vi "Query_ResonantFrequency_Sub_VI.vi"(9 "error in (no error)":errorcluster, 11 "connection ID":refnum<k5>) -> (0 "error out":errorcluster, 2 "connection ID_out":refnum<k5>, 3 "Resonant Frequencies":string)   [LabVIEW 2017]
panel:
  # "OUTPUT"
  # "INPUT"
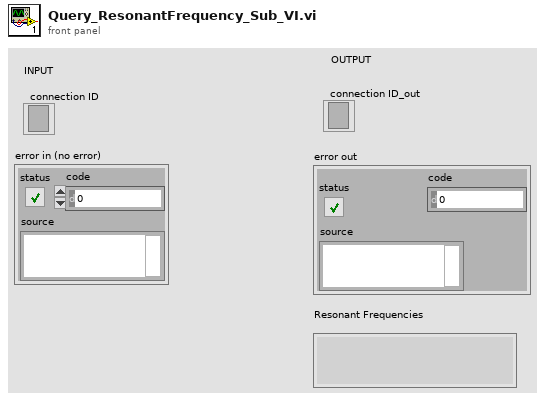
[diagram p1: front panel]
types:
  T1 = enum16{"Standard", "Buffered", "CRLF", "Immediate"}
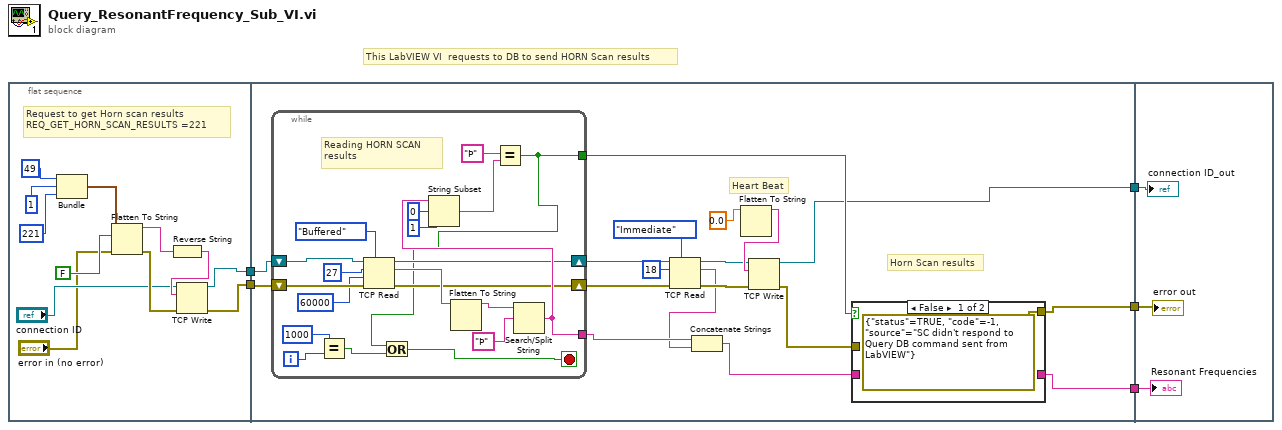
[diagram p0: block diagram]
diagram:
  # "This LabVIEW VI  requests to DB to send HORN Scan results"
  n1 = flat-sequence {
    tunnel: [w8] -> w2
    tunnel: [w7] -> w1
    tunnel: w2 -> [w33]
    tunnel: w1 -> [w32]
    tunnel: [w35] -> w5
    tunnel: [w34] -> w4
    tunnel: [w18] -> w3
    tunnel: w5 -> [w60]
    tunnel: w4 -> [w61]
    tunnel: w3 -> [w59]
    frame #0 {
      # "Request to get Horn scan results\nREQ_GET_HORN_SCAN_RESULTS =221"
      n2 = Bundle(i8 49, 1, 221) -> (w13:cluster{i8, i32, i32})  [unwired: 1 in]
      n3 = Flatten To String(anything=w13, prepend array or string size? (T)=FALSE, error in (no error)="error in (no error)") -> (data string=w12:string, error out=w16:errorcluster)  [unwired: 1 in, 1 out]
      n4 = Reverse String(1:w12) -> (0:w11:string)
      n5 = TCP Write(connection ID="connection ID", data in=w11, error in (no error)=w16) -> (connection ID out=w8:refnum<k5>, error out=w7:errorcluster)  [unwired: 1 in, 1 out]
    }
    frame #1 {
      # "Heart Beat"
      # "Horn Scan results"
      n6 = while {
        tunnel: [w37] -> w31
        tunnel: [w46] -> w21
        shift-right: [w45] -> w27
        shift-left: w33 -> [w55]
        shift-right: [w44] -> w25
        shift-left: w32 -> [w54]
        i -> [w40]
        stop <- w36 stop-if-true
        # "Reading HORN SCAN \nresults"
        n7 = Equal?(x=1000, y=w40) -> (x = y?=w38:bool)
        n8 = TCP Read(connection ID=w55, bytes to read=27, error in (no error)=w54, 7:T1."Buffered" ("mode (standard)"), 9:60000 ("timeout ms (25000)")) -> (connection ID out=w45:refnum<k5>, data out=w53:string, error out=w44:errorcluster)
        n9 = Flatten To String(anything=w53) -> (data string=w52:string)  [unwired: 3 in, 2 out]
        n10 = Search/Split String(string=w52, search string/char (-)="Þ") -> (match + rest of string=w46:string)  [unwired: 1 in, 2 out]
        n11 = String Subset(string=w46, offset (0)=0, length (rest)=1 ("length (rest)")) -> (substring=w47:string)
        n12 = Equal?(x="Þ" ("search string/char (-)"), y=w47) -> (x = y?=w37:bool)
        n13 = Or(x=w37, y=w38) -> (x .or. y?=w36:bool)
      }
      n14 = TCP Read(connection ID=w27, bytes to read=18, error in (no error)=w25, 7:T1."Immediate" ("mode (standard)")) -> (connection ID out=w26:refnum<k5>, data out=w20:string, error out=w24:errorcluster)  [unwired: 1 in]
      n15 = Concatenate Strings(w21, w20) -> (w19:string)
      n16 = Flatten To String(anything=0.0) -> (data string=w28:string)  [unwired: 3 in, 2 out]
      n17 = TCP Write(connection ID=w26, data in=w28, error in (no error)=w24) -> (connection ID out=w18:refnum<k5>, error out=w30:errorcluster)  [unwired: 1 in, 1 out]
      n18 = case shown="False" w31 {
        tunnel: [errorcluster {"status"=TRUE, "code"=-1, "source"="SC didn't respond to Query DB command sent from LabVIEW"} ("error constant") w57] -> w35
        tunnel: [_ w58] -> w34
        tunnel: w30 -> [_ w57]
        tunnel: w19 -> [_ w58]
        frame False {
        }
        frame True {
        }
      }
    }
    frame #2 {
      "error out" <- w60
      "Resonant Frequencies" <- w61
      "connection ID_out" <- w59
    }
  }
